vi "TEST - Parse XML dateTime.vi"() -> ()   [LabVIEW 2011]
panel:
  in  "current time to test":timestamp=timestamp(3550581062.8809667 s since 1904-01-01)
  out "data":timestamp
  out "x = y?":bool
  out "error out":errorcluster
  out "time stamp (local)":timestamp
  out "xml DateTime":string
  out "error out":errorcluster
  out "XML String":string
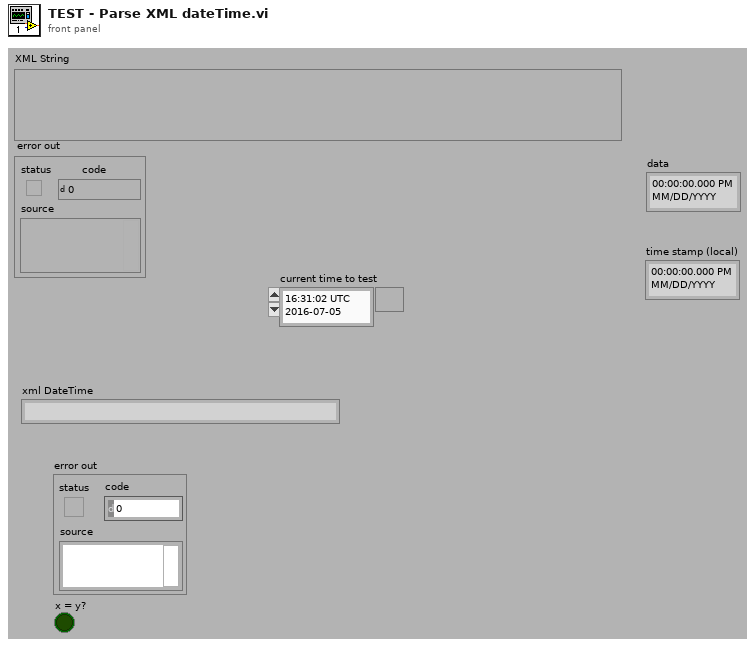
[diagram p1: front panel]
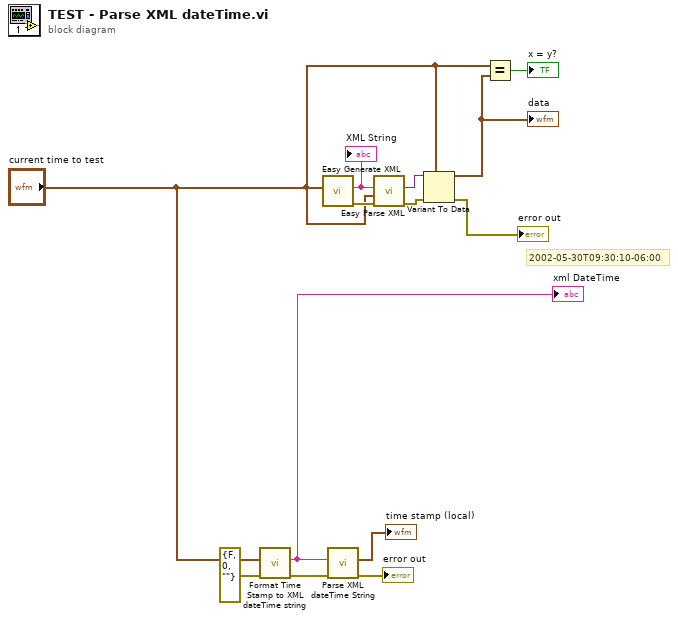
[diagram p0: block diagram]
diagram:
  # "2002-05-30T09:30:10-06:00"
  n1 = call "Format Time Stamp to XML dateTime string.vi"("error in (no error)"=errorcluster {"status"=FALSE, "code"=0, "source"=""}, "time stamp"="current time to test") -> ("error out"=w7:errorcluster, "xml dateTime string"=w9:string)  [unwired: 8 in]
  "xml DateTime" <- w9
  n2 = call "Easy Generate XML.vi"("LabVIEW Data"="current time to test") -> ("error out"=w12:errorcluster, "XML String"=w13:string)  [unwired: 9 in]
  "XML String" <- w13
  n3 = call "Parse XML dateTime String.vi"("error in (no error)"=w7, "xml dateTime string"=w9) -> ("error out"=→"error out":errorcluster, "Time Stamp"=→"time stamp (local)":timestamp)  [unwired: 8 in]
  n4 = call "Easy Parse XML.vi"("error in (no error)"=w12, "LabVIEW Data (Type)"="current time to test", "XML String"=w13) -> ("error out"=w3:errorcluster, "LabVIEW Data"=w11:variant)  [unwired: 7 in]
  n5 = Variant To Data(error in=w3, type="current time to test", Variant=w11) -> (data=w4:timestamp, error out=→"error out":errorcluster)
  "data" <- w4
  n6 = Equal?(x="current time to test", y=w4) -> (x = y?=→"x = y?":bool)
